vi "AnimationFinal.vi"() -> ()   [LabVIEW 2016]
panel:
  in  "Tab Control":enum32{"Animation "}(tab)
  out "Ring":u16(ring)
  in  "Stop":bool
  in  "Play/Pause":bool
  in  "Speed":dbl(slide) scale=0.0..1000.0
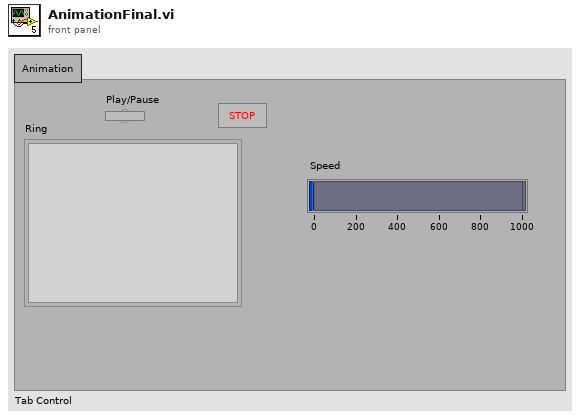
[diagram p1: front panel]
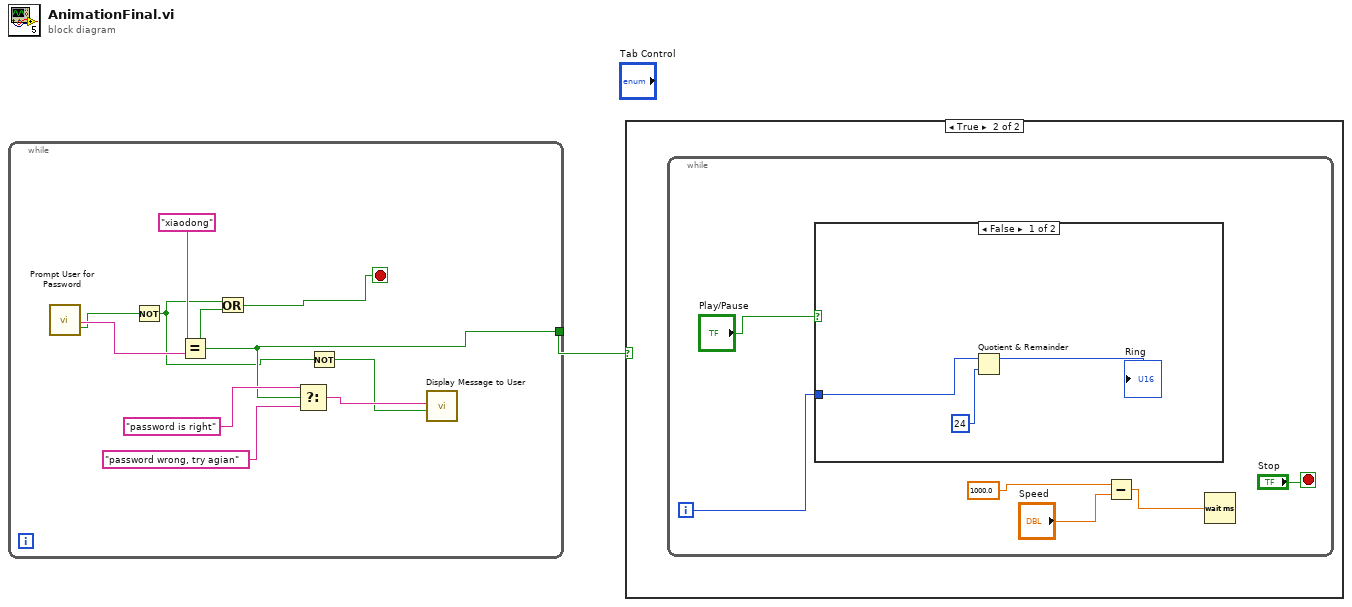
[diagram p0: block diagram]
diagram:
  n1 = while {
    tunnel: [w5] -> w1
    stop <- w4 stop-if-true
    n2 = call "Prompt User for Password"() -> ("Password"=w8:string, "OK"=w6:bool)  [unwired: 17 in, 1 out]
    n3 = Not(x=w6) -> (.not. x?=w2:bool)
    n4 = Equal?(x="xiaodong", y=w8) -> (x = y?=w5:bool)
    n5 = Or(x=w2, y=w5) -> (x .or. y?=w4:bool)
    n6 = Select(t="password is right", s=w5, f="password wrong, try agian") -> (s? t:f=w10:string)
    n7 = Not(x=w2) -> (.not. x?=w3:bool)
    n8 = call "Display Message to User"("Enable"=w3, "Message"=w10) -> ()  [unwired: 8 in, 2 out]
  }
  n9 = case shown="True" w1 {
    frame False {
    }
    frame True {
      n10 = while {
        i -> [w16]
        stop <- "Stop" stop-if-true
        n11 = case shown="False" "Play/Pause" {
          tunnel: w16 -> [w20 _]
          frame False {
            n12 = Quotient & Remainder(x=w20, y=24) -> (x-y*floor(x/y)=→"Ring":i32)  [unwired: 1 out]
          }
          frame True {
          }
        }
        n13 = Subtract(x=1000.0, y="Speed") -> (x-y=w12:dbl)
        n14 = Wait (ms)(milliseconds to wait=w12) -> ()  [unwired: 1 out]
      }
    }
  }
